vi "Mouse UP.vi"(8 "error in (no error)":errorcluster, 10 "Cell Position":T1, 11 "MCLB_Template in":refnum<class "MCLB_Template.lvclass">) -> (0 "error out":errorcluster, 3 "MCLB_Template out":refnum<class "MCLB_Template.lvclass">)   [LabVIEW 2021, in "MCLB_Template.lvclass"]
uses:
  MCLB_Template.lvclass
  <vilib>/Utility/miscctls.llb/LVRowAndColumnTypeDef.ctl
  MCLB_Template.lvclass/MCLB_Template.ctl
panel:
  out "appended array":i32[](array[numeric])
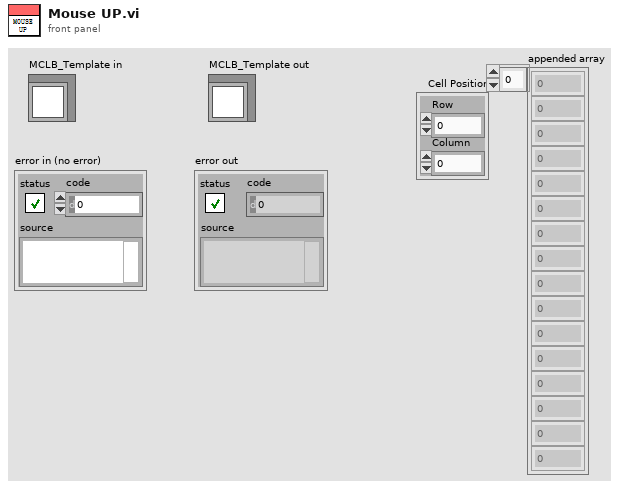
[diagram p1: front panel]
types:
  T1 = typedef "LVRowAndColumnTypeDef.ctl" = cluster{"Row":i32, "Column":i32}
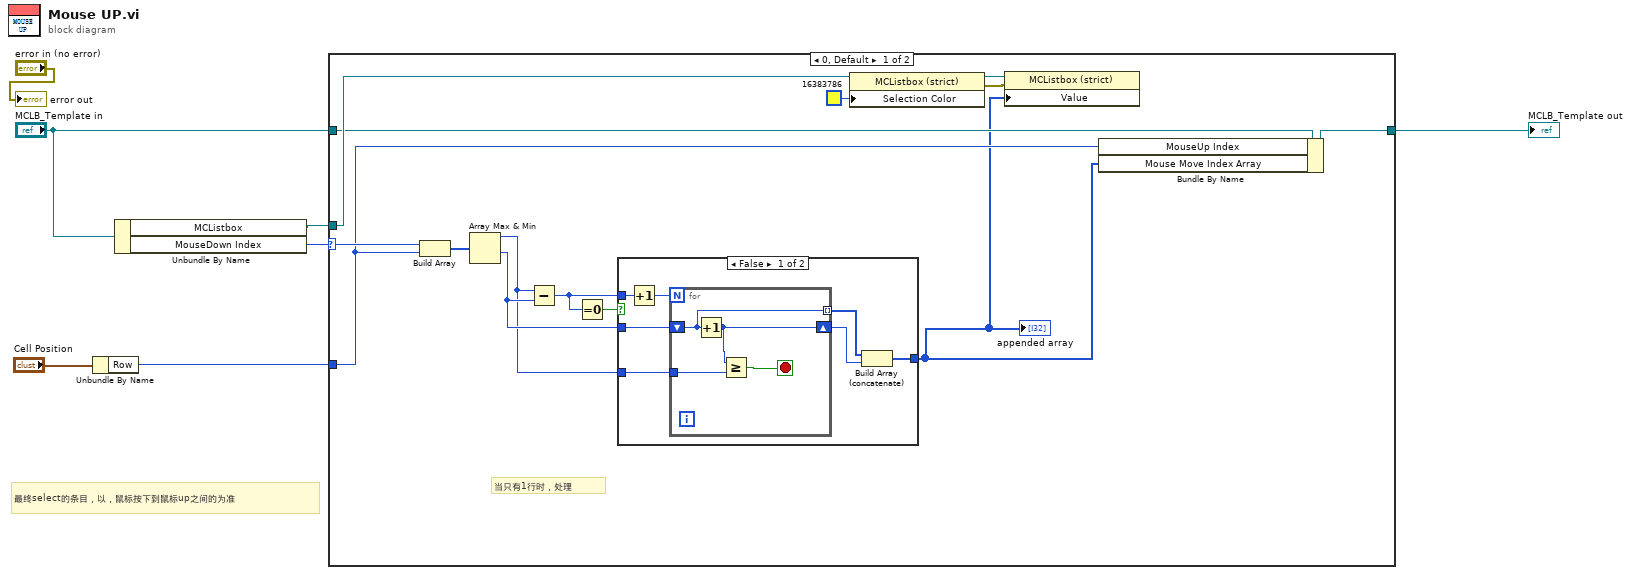
[diagram p0: block diagram]
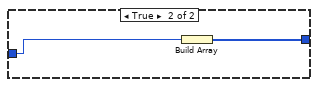
[diagram p2: hidden frame]
diagram:
  # "最终select的条目，以，鼠标按下到鼠标up之间的为准"
  n1 = Unbundle By Name("Cell Position") -> ("Row"=w5:i32)
  n2 = Unbundle By Name("MCLB_Template in") -> ("MCListbox"=w4:refnum<vi>, "MouseDown Index"=w6:i32)
  n3 = case shown="0, Default" w6 {
    selector: w6 -> [w13 _]
    tunnel: w5 -> [w9 _]
    tunnel: w4 -> [w12 _]
    tunnel: [w10 w35] -> w2
    tunnel: "MCLB_Template in" -> [w11 w35]
    frame 0, Default {
      # "当只有1行时，处理"
      n4 = Build Array(w13, w9) -> (w21:i32[])
      n5 = Array Max & Min(array=w21) -> (max value=w19:i32, min value=w20:i32)  [unwired: 2 out]
      n6 = Subtract(x=w19, y=w20) -> (x-y=w16:i32)
      n7 = Equal To 0?(x=w16) -> (x = 0?=w15:bool)
      n8 = case shown="False" w15 {
        tunnel: w20 -> [w27 _]
        tunnel: w19 -> [w26 w34]
        tunnel: w16 -> [w25 _]
        tunnel: [w22 w33] -> w8
        frame False {
          n9 = Increment(x=w25) -> (x+1=w28:i32)
          n10 = for {
            N: w28 -> [_]
            tunnel: [w29] -> w24 mode=indexing
            shift-right: [w32] -> w23
            shift-left: w27 -> [w29]
            tunnel: w26 -> [w30]
            stop <- w31 stop-if-true
            n11 = Increment(x=w29) -> (x+1=w32:i32)
            n12 = Greater Or Equal?(x=w32, y=w30) -> (x >= y?=w31:bool)
          }
          n13 = Build Array (concatenate)(w24, w23) -> (w22:i32[])
        }
        frame True {
          n14 = Build Array(w34) -> (w33:i32[])
        }
      }
      "appended array" <- w8
      n15 = property on="Property Node" class="MCListbox (strict)"(reference=w12, "Selection Color"=u32 16383786) -> (reference out=w17:refnum<vi>, error out=w18:errorcluster)  [unwired: 1 in]
      n16 = property on="Property Node" class="MCListbox (strict)"(reference=w17, error in=w18, "Value"=w8) -> ()  [unwired: 2 out]
      n17 = Bundle By Name(cluster=w11, "MouseUp Index"=w9, "Mouse Move Index Array"=w8) -> (w10:refnum<class "MCLB_Template.lvclass">)
    }
    frame -1 {
    }
  }
  "MCLB_Template out" <- w2
  "error out" <- "error in (no error)"
